vi "Init Freq list.vi"(0 "FrequencyListFile path":path, 2 "Init Amplitude [V]":dbl=0.2, 3 "error in (no error)":errorcluster) -> (7 "Frequency List":T1(array[cluster]), 10 "error out":errorcluster)   [LabVIEW 2018]
uses:
  <vilib>/Utility/file.llb/Read Delimited Spreadsheet (string).vi
panel:
  out "FrequencySteps":i32
  out "dup path":path
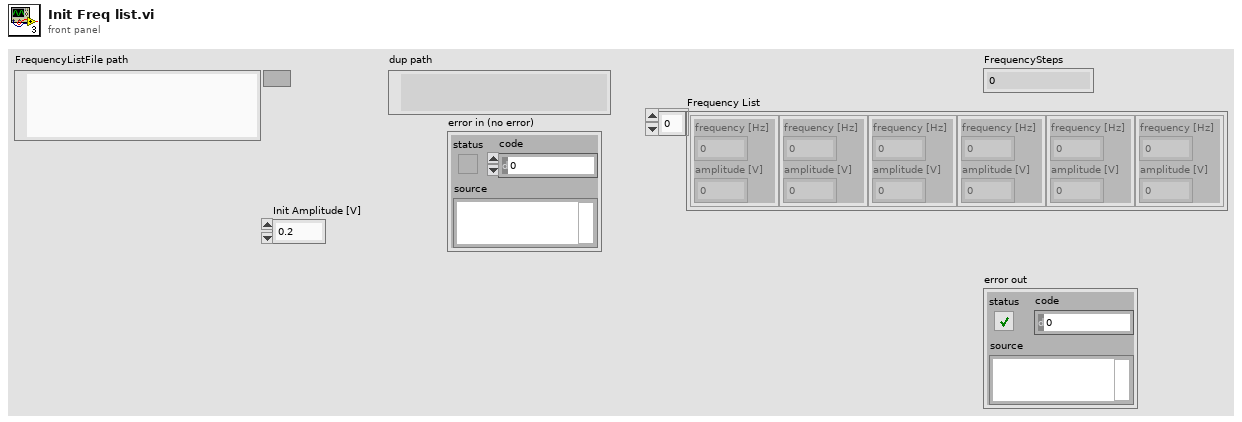
[diagram p1: front panel]
types:
  T1 = cluster{"frequency [Hz]":dbl, "amplitude [V]":dbl}[]
  T2 = cluster{"frequency [Hz]":dbl, "amplitude [V]":dbl}
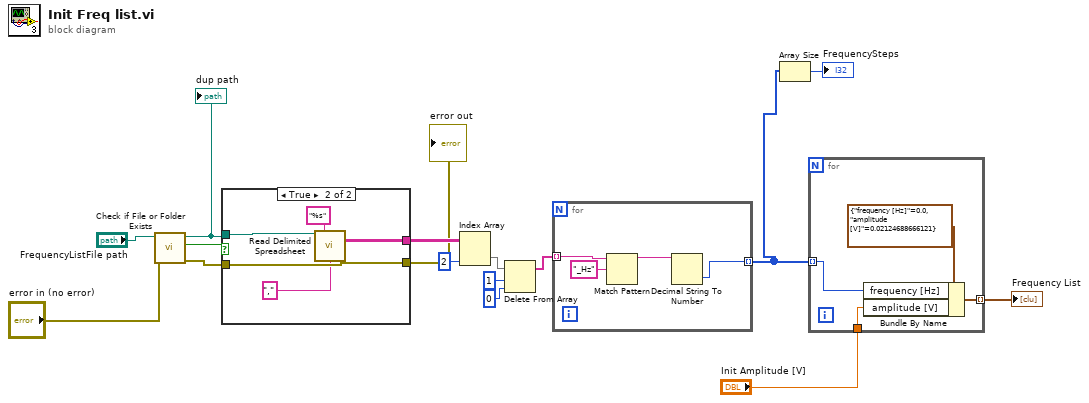
[diagram p0: block diagram]
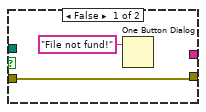
[diagram p2: hidden frame]
diagram:
  n1 = call <vilib>:"Check if File or Folder Exists.vi"("error in (no error)"="error in (no error)", "path"="FrequencyListFile path") -> ("error out"=w13:errorcluster, "file or folder exists?"=w15:bool, "dup path"=w14:path)  [unwired: 7 in]
  "dup path" <- w14
  n2 = case shown="True" w15 {
    tunnel: w14 -> [_ w22]
    tunnel: w13 -> [w18 w23]
    tunnel: [w18 w23] -> w2
    tunnel: [_ w19] -> w12
    frame False {
      n3 = One Button Dialog(message="File not fund!") -> ()  [unwired: 1 in, 1 out]
    }
    frame True {
      n4 = call-poly <vilib>:"Read Delimited Spreadsheet.vi"("file path (dialog if empty)"=w22, "format (%s)"="%s", "delimiter (\\t)"="," ("delimiter (\\t)")) -> ("all rows"=w19:string[][])  [unwired: 7 in, 5 out]
    }
  }
  "error out" <- w2
  n5 = Index Array(array=w12, index (col)=2 ("disabled index (col)")) -> (element=w10:string[])  [unwired: 1 in]
  n6 = Delete From Array(array=w10, length=1, index=0) -> (array with subset deleted=w9:string[])  [unwired: 1 out]
  n7 = for {
    tunnel: w9 -> [w27] mode=indexing
    tunnel: [w24] -> w4 mode=indexing
    n8 = Match Pattern(string=w27, regular expression="_Hz") -> (before substring=w25:string)  [unwired: 1 in, 3 out]
    n9 = Decimal String To Number(string=w25) -> (number=w24:i32)  [unwired: 2 in, 1 out]
  }
  n10 = Array Size(array=w4) -> (size(s)=→"FrequencySteps":i32)
  n11 = for {
    tunnel: w4 -> [w31] mode=indexing
    tunnel: "Init Amplitude [V]" -> [w30]
    tunnel: [w28] -> w7 mode=indexing
    n12 = Bundle By Name(cluster=T2 {"frequency [Hz]"=0.0, "amplitude [V]"=0.02124688666121} ("tone settings 2"), "frequency [Hz]"=w31, "amplitude [V]"=w30) -> (w28:T2)
  }
  "Frequency List" <- w7
